vi "get_weather.vi"(4 "Weather Index":u32, 5 "Weather Profiles":refnum<vi>, 6 "error in":errorcluster, 7 "External Weather Control":bool, 9 "simx in":T2={"Config"={"Trajectory"={"Number of frames"=0, "Frame number"=0, "Trajectory"=""}, "Weather"={"id"=""}}, "Connections"={"Simulator Connection"=refnum, "server_ip"="127.0.0.1", "Port"=0, "Sensor connections"=[]}, "Map"={"lanes"={"x"=[], "y"=[], "z"=[]}, "StartPosition"={"start_points"={"locations"=[], "rotations"=[], "type"=[]}, "StartRotation"=[], "StartLocation"=[]}, "Draw Map Size"={"Width"=0, "Height"=0}, "DrawArea"={"min_Y"=0.0, "min_X"=0.0, "Scale X"=0.0, "Scale Y"=0.0}, "Map"=bytes[0], "Map Geojson"=""}}) -> (0 "error out":errorcluster, 1 "Weather Profiles":T9(array[cluster]), 2 "Id":string, 3 "simx out":T2={"Config"={"Trajectory"={"Number of frames"=0, "Frame number"=0, "Trajectory"=""}, "Weather"={"id"=""}}, "Connections"={"Simulator Connection"=refnum, "server_ip"="127.0.0.1", "Port"=0, "Sensor connections"=[]}, "Map"={"lanes"={"x"=[], "y"=[], "z"=[]}, "StartPosition"={"start_points"={"locations"=[], "rotations"=[], "type"=[]}, "StartRotation"=[], "StartLocation"=[]}, "Draw Map Size"={"Width"=0, "Height"=0}, "DrawArea"={"min_Y"=0.0, "min_X"=0.0, "Scale X"=0.0, "Scale Y"=0.0}, "Map"=bytes[0], "Map Geojson"=""}})   [LabVIEW 2025]
doc: "Obtains the weather configuration from a file and populates a cluster with the configuration."
uses:
  controls/simx_connection.ctl
  controls/config.ctl
  controls/trajectory.ctl
  controls/weather.ctl
  controls/connections.ctl
  controls/start_points.ctl
  <vilib>/Utility/miscctls.llb/LVBoundsTypeDef.ctl
  tools/simx_common.vi
panel:
  in  "Cluster":T1
  in  "Weather Configuration":string="{\n \"descriptions\": [\n  {\n   \"CloudColor\": {\n    \"A\": 1.0,\n    \"B\": 1.0,\n    \"G\": 0.9190000295639038,\n    \"R\": 0.8557999730110168\n   },\n   \"CloudOpacity\": 1.1399999856948853,\n   \"Day\": 1,\n   \"FogCutoffDistance\": 0.0,\n   \"FogDensity\": 0.0,\n   \"FogHeightFalloff\": 0.20000000298023224,\n   \"FogInscatteringColor\": {\n    \"A\": 1.0,\n    \"B\": 1.0,\n    \"G\": 0.6380000114440918,\n    \"R\": 0.4449999928474426\n   },\n   \"FogMaxOpacity\": 1.0,\n   \"FogStartDistance\": 0.0,\n   \"HorizonColor\": {\n    \"A\": 1.0,\n    \"B\": 1.0,\n    \"G\": 0.8622000217437744,\n    \"R\": 0.6599000096321106\n   },\n   \"HorizonFalloff\": 10.0,\n   \"Hours\": 12,\n   \"IsDaylightSavingTime\": true,\n   \"Latitude\": 30.237119674682617,\n   \"Longitude\": -97.66307067871094,\n   \"Minutes\": 0,\n   \"Month\": 6,\n   \"NorthOffset\": 0.0,\n   \"OverallSkyColor\": {\n    \"A\": 1.0,\n    \"B\": 1.0,\n    \"G\": 1.0,\n    \"R\": 1.0\n   },\n   \"OverideTimeBasedSunAngle\": false,\n   \"PrecipitationAccumulation\": 0.0,\n   \"PrecipitationAmount\": 0.0,\n   \"PrecipitationType\": \"Rain\",\n   \"SecondFogDensity\": 0.0,\n   \"SecondFogHeightFalloff\": 0.20000000298023224,\n   \"SecondFogHeightOffset\": 0.0,\n   \"Seconds\": 0,\n   \"SkyLightColor\": {\n    \"A\": 0.0,\n    \"B\": 0.1412999927997589,\n    \"G\": 0.1851000040769577,\n    \"R\": 0.19499999284744263\n   },\n   \"SkyLightIntensity\": 1.0,\n   \"StarBrightness\": 3.0,\n   \"SunAzimuthAngle\": 45.0,\n   \"SunBrightness\": 3000.0,\n   \"SunDirectionalLightColor\": {\n    \"A\": 1.0,\n    \"B\": 194.0,\n    \"G\": 239.0,\n    \"R\": 255.0\n   },\n   \"SunDirectionalLightIntensity\": 3.0,\n   \"SunPolarAngle\": 45.0,\n   \"TimeZone\": -5.0,\n   \"WindAngle\": 0.0,\n   \"WindIntensity\": 20.0,\n   \"Year\": 2022,\n   \"ZenithColor\": {\n    \"A\": 1.0,\n    \"B\": 0.29499998688697815,\n    \"G\": 0.10920000076293945,\n    \"R\": 0.03400000184774399\n   },\n   \"bPrecipitation\": false,\n   \"bWind\": false,\n   \"id\": \"Default\"\n  },\n  {\n   \"CloudColor\": {\n    \"A\": 1.0,\n    \"B\": 1.0,\n    \"G\": 0.9190000295639038,\n    \"R\": 0.8557999730110168\n   },\n   \"CloudOpacity\": 0.4285709857940674,\n   \"Day\": 1,\n   \"FogCutoffDistance\": 0.0,\n   \"FogDensity\": 0.007000000216066837,\n   \"FogHeightFalloff\": 1.0671329498291016,\n   \"FogInscatteringColor\": {\n    \"A\": 1.0,\n    \"B\": 1.0,\n    \"G\": 0.6380000114440918,\n    \"R\": 0.4449999928474426\n   },\n   \"FogMaxOpacity\": 1.0,\n   \"FogStartDistance\": 0.0,\n   \"HorizonColor\": {\n    \"A\": 1.0,\n    \"B\": 1.0,\n    \"G\": 0.8622000217437744,\n    \"R\": 0.6599000096321106\n   },\n   \"HorizonFalloff\": 14.28571605682373,\n   \"Hours\": 12,\n   \"IsDaylightSavingTime\": true,\n   \"Latitude\": 30.237119674682617,\n   \"Longitude\": -97.66307067871094,\n   \"Minutes\": 0,\n   \"Month\": 6,\n   \"NorthOffset\": 0.0,\n   \"OverallSkyColor\": {\n    \"A\": 1.0,\n    \"B\": 1.0,\n    \"G\": 1.0,\n    \"R\": 1.0\n   },\n   \"OverideTimeBasedSunAngle\": false,\n   \"PrecipitationAccumulation\": 0.0,\n   \"PrecipitationAmount\": 0.0,\n   \"PrecipitationType\": \"Rain\",\n   \"SecondFogDensity\": 0.0,\n   \"SecondFogHeightFalloff\": 0.3436860144138336,\n   \"SecondFogHeightOffset\": -0.12381000071763992,\n   \"Seconds\": 0,\n   \"SkyLightColor\": {\n    \"A\": 0.0,\n    \"B\": 0.1412999927997589,\n    \"G\": 0.1851000040769577,\n    \"R\": 0.19499999284744263\n   },\n   \"SkyLightIntensity\": 0.5,\n   \"StarBrightness\": 3.0,\n   \"SunAzimuthAngle\": 45.0,\n   \"SunBrightness\": 3000.0,\n   \"SunDirectionalLightColor\": {\n    \"A\": 1.0,\n    \"B\": 1.0,\n    \"G\": 1.0,\n    \"R\": 1.0\n   },\n   \"SunDirectionalLightIntensity\": 3.0,\n   \"SunPolarAngle\": 45.0,\n   \"TimeZone\": -5.0,\n   \"WindAngle\": 0.0,\n   \"WindIntensity\": 20.0,\n   \"Year\": 2022,\n   \"ZenithColor\": {\n    \"A\": 1.0,\n    \"B\": 0.29499998688697815,\n    \"G\": 0.10920000076293945,\n    \"R\": 0.03400000184774399\n   },\n   \"bPrecipitation\": false,\n   \"bWind\": false,\n   \"id\": \"ClearNoon\"\n  },\n  {\n   \"CloudColor\": {\n    \"A\": 1.0,\n    \"B\": 0.05208300054073334,\n    \"G\": 0.05208300054073334,\n    \"R\": 0.05208300054073334\n   },\n   \"CloudOpacity\": 4.0,\n   \"Day\": 1,\n   \"FogCutoffDistance\": 0.0,\n   \"FogDensity\": 0.009999999776482582,\n   \"FogHeightFalloff\": 0.20000000298023224,\n   \"FogInscatteringColor\": {\n    \"A\": 1.0,\n    \"B\": 0.49479201436042786,\n    \"G\": 0.47966399788856506,\n    \"R\": 0.4715990126132965\n   },\n   \"FogMaxOpacity\": 1.0,\n   \"FogStartDistance\": 0.0,\n   \"HorizonColor\": {\n    \"A\": 1.0,\n    \"B\": 0.20000000298023224,\n    \"G\": 0.18744300305843353,\n    \"R\": 0.16899999976158142\n   },\n   \"HorizonFalloff\": 0.0,\n   \"Hours\": 14,\n   \"IsDaylightSavingTime\": true,\n   \"Latitude\": 30.237119674682617,\n   \"Longitude\": -97.66307067871094,\n   \"Minutes\": 0,\n   \"Month\": 6,\n   \"NorthOffset\": 0.0,\n   \"OverallSkyColor\": {\n    \"A\": 1.0,\n    \"B\": 1.0,\n    \"G\": 1.0,\n    \"R\": 1.0\n   },\n   \"OverideTimeBasedSunAngle\": false,\n   \"PrecipitationAccumulation\": 0.0,\n   \"PrecipitationAmount\": 0.0,\n   \"PrecipitationType\": \"Rain\",\n   \"SecondFogDensity\": 0.0,\n   \"SecondFogHeightFalloff\": 0.20000000298023224,\n   \"SecondFogHeightOffset\": 0.0,\n   \"Seconds\": 0,\n   \"SkyLightColor\": {\n    \"A\": 0.0,\n    \"B\": 0.14499999582767487,\n    \"G\": 0.10680299997329712,\n    \"R\": 0.1008870005607605\n   },\n   \"SkyLightIntensity\": 0.5,\n   \"StarBrightness\": 3.0,\n   \"SunAzimuthAngle\": 45.0,\n   \"SunBrightness\": 3000.0,\n   \"SunDirectionalLightColor\": {\n    \"A\": 1.0,\n    \"B\": 0.25520798563957214,\n    \"G\": 0.25520798563957214,\n    \"R\": 0.25520798563957214\n   },\n   \"SunDirectionalLightIntensity\": 3.0,\n   \"SunPolarAngle\": 45.0,\n   \"TimeZone\": -5.0,\n   \"WindAngle\": 0.0,\n   \"WindIntensity\": 20.0,\n   \"Year\": 2022,\n   \"ZenithColor\": {\n    \"A\": 1.0,\n    \"B\": 0.29499998688697815,\n    \"G\": 0.1812479943037033,\n    \"R\": 0.13520799577236176\n   },\n   \"bPrecipitation\": false,\n   \"bWind\": false,\n   \"id\": \"CloudyNoon\"\n  },\n  {\n   \"CloudColor\": {\n    \"A\": 1.0,\n    \"B\": 0.1899999976158142,\n    \"G\": 0.15923500061035156,\n    \"R\": 0.14362700283527374\n   },\n   \"CloudOpacity\": 1.5714290142059326,\n   \"Day\": 1,\n   \"FogCutoffDistance\": 0.0,\n   \"FogDensity\": 0.005237999837845564,\n   \"FogHeightFalloff\": 0.20000000298023224,\n   \"FogInscatteringColor\": {\n    \"A\": 1.0,\n    \"B\": 1.0,\n    \"G\": 0.6380000114440918,\n    \"R\": 0.4449999928474426\n   },\n   \"FogMaxOpacity\": 0.028571000322699547,\n   \"FogStartDistance\": 0.0,\n   \"HorizonColor\": {\n    \"A\": 1.0,\n    \"B\": 0.6299999952316284,\n    \"G\": 0.5904449820518494,\n    \"R\": 0.5323500037193298\n   },\n   \"HorizonFalloff\": 10.476192474365234,\n   \"Hours\": 12,\n   \"IsDaylightSavingTime\": true,\n   \"Latitude\": 30.237119674682617,\n   \"Longitude\": -97.66307067871094,\n   \"Minutes\": 0,\n   \"Month\": 6,\n   \"NorthOffset\": 0.0,\n   \"OverallSkyColor\": {\n    \"A\": 1.0,\n    \"B\": 0.5181000232696533,\n    \"G\": 0.6304129958152771,\n    \"R\": 0.6600000262260437\n   },\n   \"OverideTimeBasedSunAngle\": false,\n   \"PrecipitationAccumulation\": 28.57143211364746,\n   \"PrecipitationAmount\": 0.0,\n   \"PrecipitationType\": \"Rain\",\n   \"SecondFogDensity\": 0.001429000054486096,\n   \"SecondFogHeightFalloff\": 2.0,\n   \"SecondFogHeightOffset\": 0.3131600022315979,\n   \"Seconds\": 0,\n   \"SkyLightColor\": {\n    \"A\": 0.0,\n    \"B\": 0.07559999823570251,\n    \"G\": 0.12014999985694885,\n    \"R\": 0.13500000536441803\n   },\n   \"SkyLightIntensity\": 1.0,\n   \"StarBrightness\": 3.0,\n   \"SunAzimuthAngle\": 45.0,\n   \"SunBrightness\": 0.0,\n   \"SunDirectionalLightColor\": {\n    \"A\": 1.0,\n    \"B\": 1.0,\n    \"G\": 1.0,\n    \"R\": 1.0\n   },\n   \"SunDirectionalLightIntensity\": 3.0,\n   \"SunPolarAngle\": 45.0,\n   \"TimeZone\": -5.0,\n   \"WindAngle\": 0.0,\n   \"WindIntensity\": 20.0,\n   \"Year\": 2022,\n   \"ZenithColor\": {\n    \"A\": 1.0,\n    \"B\": 0.29499998688697815,\n    \"G\": 0.10920000076293945,\n    \"R\": 0.03400000184774399\n   },\n   \"bPrecipitation\": true,\n   \"bWind\": false,\n   \"id\": \"WetNoon\"\n  },\n  {\n   \"CloudColor\": {\n    \"A\": 1.0,\n    \"B\": 0.27164098620414734,\n    \"G\": 0.3050000071525574,\n    \"R\": 0.2995159924030304\n   },\n   \"CloudOpacity\": 1.0,\n   \"Day\": 1,\n   \"FogCutoffDistance\": 0.0,\n   \"FogDensity\": 0.009523999877274036,\n   \"FogHeightFalloff\": 0.20000000298023224,\n   \"FogInscatteringColor\": {\n    \"A\": 1.0,\n    \"B\": 1.0,\n    \"G\": 0.8581939935684204,\n    \"R\": 0.548704981803894\n   },\n   \"FogMaxOpacity\": 1.0,\n   \"FogStartDistance\": 0.0,\n   \"HorizonColor\": {\n    \"A\": 1.0,\n    \"B\": 0.0,\n    \"G\": 0.0,\n    \"R\": 0.0\n   },\n   \"HorizonFalloff\": 3.0,\n   \"Hours\": 12,\n   \"IsDaylightSavingTime\": true,\n   \"Latitude\": 30.237119674682617,\n   \"Longitude\": -97.66307067871094,\n   \"Minutes\": 0,\n   \"Month\": 6,\n   \"NorthOffset\": 0.0,\n   \"OverallSkyColor\": {\n    \"A\": 1.0,\n    \"B\": 0.5181000232696533,\n    \"G\": 0.6304129958152771,\n    \"R\": 0.6600000262260437\n   },\n   \"OverideTimeBasedSunAngle\": false,\n   \"PrecipitationAccumulation\": 47.70600128173828,\n   \"PrecipitationAmount\": 0.0,\n   \"PrecipitationType\": \"Rain\",\n   \"SecondFogDensity\": 0.0,\n   \"SecondFogHeightFalloff\": 0.20000000298023224,\n   \"SecondFogHeightOffset\": 0.0,\n   \"Seconds\": 0,\n   \"SkyLightColor\": {\n    \"A\": 0.0,\n    \"B\": 0.1267089992761612,\n    \"G\": 0.13369999825954437,\n    \"R\": 0.140625\n   },\n   \"SkyLightIntensity\": 1.0,\n   \"StarBrightness\": 3.0,\n   \"SunAzimuthAngle\": 174.0,\n   \"SunBrightness\": 0.0,\n   \"SunDirectionalLightColor\": {\n    \"A\": 1.0,\n    \"B\": 0.20507900416851044,\n    \"G\": 0.30498701333999634,\n    \"R\": 0.2874409854412079\n   },\n   \"SunDirectionalLightIntensity\": 1.8350000381469727,\n   \"SunPolarAngle\": 174.0,\n   \"TimeZone\": -5.0,\n   \"WindAngle\": 0.0,\n   \"WindIntensity\": 20.0,\n   \"Year\": 2018,\n   \"ZenithColor\": {\n    \"A\": 1.0,\n    \"B\": 1.0,\n    \"G\": 1.0,\n    \"R\": 1.0\n   },\n   \"bPrecipitation\": true,\n   \"bWind\": false,\n   \"id\": \"WetCloudyNoon\"\n  },\n  {\n   \"CloudColor\": {\n    \"A\": 1.0,\n    \"B\": 0.05000000074505806,\n    \"G\": 0.04594999924302101,\n    \"R\": 0.042789001017808914\n   },\n   \"CloudOpacity\": 1.0,\n   \"Day\": 1,\n   \"FogCutoffDistance\": 0.0,\n   \"FogDensity\": 0.008570999838411808,\n   \"FogHeightFalloff\": 0.20000000298023224,\n   \"FogInscatteringColor\": {\n    \"A\": 1.0,\n    \"B\": 0.4889959990978241,\n    \"G\": 0.6769369840621948,\n    \"R\": 0.7395830154418945\n   },\n   \"FogMaxOpacity\": 1.0,\n   \"FogStartDistance\": 0.0,\n   \"HorizonColor\": {\n    \"A\": 1.0,\n    \"B\": 0.20000000298023224,\n    \"G\": 0.18744300305843353,\n    \"R\": 0.16899999976158142\n   },\n   \"HorizonFalloff\": 3.0,\n   \"Hours\": 12,\n   \"IsDaylightSavingTime\": true,\n   \"Latitude\": 30.237119674682617,\n   \"Longitude\": -97.66307067871094,\n   \"Minutes\": 0,\n   \"Month\": 6,\n   \"NorthOffset\": 0.0,\n   \"OverallSkyColor\": {\n    \"A\": 1.0,\n    \"B\": 1.0,\n    \"G\": 1.0,\n    \"R\": 1.0\n   },\n   \"OverideTimeBasedSunAngle\": false,\n   \"PrecipitationAccumulation\": 50.0,\n   \"PrecipitationAmount\": 40.0,\n   \"PrecipitationType\": \"Rain\",\n   \"SecondFogDensity\": 0.0,\n   \"SecondFogHeightFalloff\": 0.20000000298023224,\n   \"SecondFogHeightOffset\": 0.0,\n   \"Seconds\": 0,\n   \"SkyLightColor\": {\n    \"A\": 0.0,\n    \"B\": 0.17000000178813934,\n    \"G\": 0.12155699729919434,\n    \"R\": 0.1198820024728775\n   },\n   \"SkyLightIntensity\": 1.0,\n   \"StarBrightness\": 3.0,\n   \"SunAzimuthAngle\": 45.0,\n   \"SunBrightness\": 3000.0,\n   \"SunDirectionalLightColor\": {\n    \"A\": 1.0,\n    \"B\": 1.0,\n    \"G\": 1.0,\n    \"R\": 1.0\n   },\n   \"SunDirectionalLightIntensity\": 3.0,\n   \"SunPolarAngle\": 45.0,\n   \"TimeZone\": -5.0,\n   \"WindAngle\": -80.0,\n   \"WindIntensity\": 40.0,\n   \"Year\": 2022,\n   \"ZenithColor\": {\n    \"A\": 1.0,\n    \"B\": 0.3700000047683716,\n    \"G\": 0.3700000047683716,\n    \"R\": 0.3700000047683716\n   },\n   \"bPrecipitation\": true,\n   \"bWind\": true,\n   \"id\": \"MidRainyNoon\"\n  },\n  {\n   \"CloudColor\": {\n    \"A\": 1.0,\n    \"B\": 0.046875,\n    \"G\": 0.04307800158858299,\n    \"R\": 0.04011499881744385\n   },\n   \"CloudOpacity\": 1.0,\n   \"Day\": 1,\n   \"FogCutoffDistance\": 0.0,\n   \"FogDensity\": 0.0042860000394284725,\n   \"FogHeightFalloff\": 0.4007999897003174,\n   \"FogInscatteringColor\": {\n    \"A\": 1.0,\n    \"B\": 1.0,\n    \"G\": 0.6380000114440918,\n    \"R\": 0.4449999928474426\n   },\n   \"FogMaxOpacity\": 0.5904759764671326,\n   \"FogStartDistance\": 0.0,\n   \"HorizonColor\": {\n    \"A\": 1.0,\n    \"B\": 0.11458300054073334,\n    \"G\": 0.10738900303840637,\n    \"R\": 0.09682299941778183\n   },\n   \"HorizonFalloff\": 3.0,\n   \"Hours\": 12,\n   \"IsDaylightSavingTime\": true,\n   \"Latitude\": 30.237119674682617,\n   \"Longitude\": -97.66307067871094,\n   \"Minutes\": 0,\n   \"Month\": 6,\n   \"NorthOffset\": 0.0,\n   \"OverallSkyColor\": {\n    \"A\": 1.0,\n    \"B\": 0.23455099761486053,\n    \"G\": 0.18782100081443787,\n    \"R\": 0.15592600405216217\n   },\n   \"OverideTimeBasedSunAngle\": false,\n   \"PrecipitationAccumulation\": 87.24800109863281,\n   \"PrecipitationAmount\": 80.0,\n   \"PrecipitationType\": \"Rain\",\n   \"SecondFogDensity\": 0.010475999675691128,\n   \"SecondFogHeightFalloff\": 1.1899809837341309,\n   \"SecondFogHeightOffset\": 0.6190469861030579,\n   \"Seconds\": 0,\n   \"SkyLightColor\": {\n    \"A\": 0.0,\n    \"B\": 0.18000000715255737,\n    \"G\": 0.12870700657367706,\n    \"R\": 0.1269340068101883\n   },\n   \"SkyLightIntensity\": 1.0,\n   \"StarBrightness\": 3.0,\n   \"SunAzimuthAngle\": 45.0,\n   \"SunBrightness\": 0.0,\n   \"SunDirectionalLightColor\": {\n    \"A\": 1.0,\n    \"B\": 0.203125,\n    \"G\": 0.1996610015630722,\n    \"R\": 0.1996610015630722\n   },\n   \"SunDirectionalLightIntensity\": 3.0,\n   \"SunPolarAngle\": 45.0,\n   \"TimeZone\": -5.0,\n   \"WindAngle\": -60.0,\n   \"WindIntensity\": 39.0476188659668,\n   \"Year\": 2022,\n   \"ZenithColor\": {\n    \"A\": 1.0,\n    \"B\": 0.5799999833106995,\n    \"G\": 0.5799999833106995,\n    \"R\": 0.5799999833106995\n   },\n   \"bPrecipitation\": true,\n   \"bWind\": true,\n   \"id\": \"HardRainNoon\"\n  },\n  {\n   \"CloudColor\": {\n    \"A\": 1.0,\n    \"B\": 0.18229199945926666,\n    \"G\": 0.1675260066986084,\n    \"R\": 0.1560010015964508\n   },\n   \"CloudOpacity\": 1.0,\n   \"Day\": 1,\n   \"FogCutoffDistance\": 0.0,\n   \"FogDensity\": 0.03333299979567528,\n   \"FogHeightFalloff\": 0.20000000298023224,\n   \"FogInscatteringColor\": {\n    \"A\": 1.0,\n    \"B\": 0.375,\n    \"G\": 0.3648090064525604,\n    \"R\": 0.359375\n   },\n   \"FogMaxOpacity\": 1.0,\n   \"FogStartDistance\": 0.0,\n   \"HorizonColor\": {\n    \"A\": 1.0,\n    \"B\": 0.20000000298023224,\n    \"G\": 0.18744300305843353,\n    \"R\": 0.16899999976158142\n   },\n   \"HorizonFalloff\": 3.0,\n   \"Hours\": 10,\n   \"IsDaylightSavingTime\": true,\n   \"Latitude\": 30.237119674682617,\n   \"Longitude\": -97.66307067871094,\n   \"Minutes\": 0,\n   \"Month\": 6,\n   \"NorthOffset\": 0.0,\n   \"OverallSkyColor\": {\n    \"A\": 1.0,\n    \"B\": 1.0,\n    \"G\": 1.0,\n    \"R\": 1.0\n   },\n   \"OverideTimeBasedSunAngle\": false,\n   \"PrecipitationAccumulation\": 61.926998138427734,\n   \"PrecipitationAmount\": 10.550000190734863,\n   \"PrecipitationType\": \"Rain\",\n   \"SecondFogDensity\": 0.018571000546216965,\n   \"SecondFogHeightFalloff\": 0.20000000298023224,\n   \"SecondFogHeightOffset\": 0.0,\n   \"Seconds\": 0,\n   \"SkyLightColor\": {\n    \"A\": 0.0,\n    \"B\": 0.07291699945926666,\n    \"G\": 0.07291699945926666,\n    \"R\": 0.07291699945926666\n   },\n   \"SkyLightIntensity\": 0.5,\n   \"StarBrightness\": 3.0,\n   \"SunAzimuthAngle\": 45.0,\n   \"SunBrightness\": 3000.0,\n   \"SunDirectionalLightColor\": {\n    \"A\": 1.0,\n    \"B\": 1.0,\n    \"G\": 1.0,\n    \"R\": 1.0\n   },\n   \"SunDirectionalLightIntensity\": 1.5,\n   \"SunPolarAngle\": 45.0,\n   \"TimeZone\": -5.0,\n   \"WindAngle\": 20.0,\n   \"WindIntensity\": 10.0,\n   \"Year\": 2022,\n   \"ZenithColor\": {\n    \"A\": 1.0,\n    \"B\": 0.0,\n    \"G\": 0.0,\n    \"R\": 0.0\n   },\n   \"bPrecipitation\": true,\n   \"bWind\": true,\n   \"id\": \"SoftRainNoon\"\n  },\n  {\n   \"CloudColor\": {\n    \"A\": 1.0,\n    \"B\": 0.08333300054073334,\n    \"G\": 0.5042790174484253,\n    \"R\": 1.0\n   },\n   \"CloudOpacity\": 0.5714290142059326,\n   \"Day\": 1,\n   \"FogCutoffDistance\": 0.0,\n   \"FogDensity\": 0.003000000026077032,\n   \"FogHeightFalloff\": 0.20000000298023224,\n   \"FogInscatteringColor\": {\n    \"A\": 1.0,\n    \"B\": 0.4279409945011139,\n    \"G\": 0.7066850066184998,\n    \"R\": 0.8470590114593506\n   },\n   \"FogMaxOpacity\": 1.0,\n   \"FogStartDistance\": 2800.0,\n   \"HorizonColor\": {\n    \"A\": 1.0,\n    \"B\": 0.04664900153875351,\n    \"G\": 0.2190060019493103,\n    \"R\": 0.7450000047683716\n   },\n   \"HorizonFalloff\": 3.0,\n   \"Hours\": 19,\n   \"IsDaylightSavingTime\": true,\n   \"Latitude\": 30.237119674682617,\n   \"Longitude\": -97.66307067871094,\n   \"Minutes\": 0,\n   \"Month\": 6,\n   \"NorthOffset\": 0.0,\n   \"OverallSkyColor\": {\n    \"A\": 1.0,\n    \"B\": 1.0,\n    \"G\": 1.0,\n    \"R\": 1.0\n   },\n   \"OverideTimeBasedSunAngle\": false,\n   \"PrecipitationAccumulation\": 0.0,\n   \"PrecipitationAmount\": 0.0,\n   \"PrecipitationType\": \"Rain\",\n   \"SecondFogDensity\": 0.0020000000949949026,\n   \"SecondFogHeightFalloff\": 0.6000000238418579,\n   \"SecondFogHeightOffset\": 0.0,\n   \"Seconds\": 0,\n   \"SkyLightColor\": {\n    \"A\": 0.0,\n    \"B\": 0.109375,\n    \"G\": 0.07472400367259979,\n    \"R\": 0.07621999830007553\n   },\n   \"SkyLightIntensity\": 1.0,\n   \"StarBrightness\": 3.0,\n   \"SunAzimuthAngle\": 45.0,\n   \"SunBrightness\": 3000.0,\n   \"SunDirectionalLightColor\": {\n    \"A\": 1.0,\n    \"B\": 0.17010000348091125,\n    \"G\": 0.3474699854850769,\n    \"R\": 0.8100000023841858\n   },\n   \"SunDirectionalLightIntensity\": 3.0,\n   \"SunPolarAngle\": 45.0,\n   \"TimeZone\": -5.0,\n   \"WindAngle\": 0.0,\n   \"WindIntensity\": 20.0,\n   \"Year\": 2022,\n   \"ZenithColor\": {\n    \"A\": 1.0,\n    \"B\": 0.10499999672174454,\n    \"G\": 0.04410000145435333,\n    \"R\": 0.04637499898672104\n   },\n   \"bPrecipitation\": false,\n   \"bWind\": false,\n   \"id\": \"ClearSunset\"\n  },\n  {\n   \"CloudColor\": {\n    \"A\": 1.0,\n    \"B\": 0.13456499576568604,\n    \"G\": 0.20229600369930267,\n    \"R\": 0.5208330154418945\n   },\n   \"CloudOpacity\": 1.4285720586776733,\n   \"Day\": 1,\n   \"FogCutoffDistance\": 0.0,\n   \"FogDensity\": 0.0009519999730400741,\n   \"FogHeightFalloff\": 0.20000000298023224,\n   \"FogInscatteringColor\": {\n    \"A\": 1.0,\n    \"B\": 0.4463469982147217,\n    \"G\": 0.5565620064735413,\n    \"R\": 1.0\n   },\n   \"FogMaxOpacity\": 1.0,\n   \"FogStartDistance\": 0.0,\n   \"HorizonColor\": {\n    \"A\": 1.0,\n    \"B\": 0.09927500039339066,\n    \"G\": 0.18896199762821198,\n    \"R\": 1.0\n   },\n   \"HorizonFalloff\": 3.5,\n   \"Hours\": 19,\n   \"IsDaylightSavingTime\": true,\n   \"Latitude\": 30.237119674682617,\n   \"Longitude\": -97.66307067871094,\n   \"Minutes\": 0,\n   \"Month\": 6,\n   \"NorthOffset\": 0.0,\n   \"OverallSkyColor\": {\n    \"A\": 1.0,\n    \"B\": 0.4099999964237213,\n    \"G\": 0.4099999964237213,\n    \"R\": 0.4099999964237213\n   },\n   \"OverideTimeBasedSunAngle\": false,\n   \"PrecipitationAccumulation\": 0.0,\n   \"PrecipitationAmount\": 0.0,\n   \"PrecipitationType\": \"Rain\",\n   \"SecondFogDensity\": 0.0,\n   \"SecondFogHeightFalloff\": 0.20000000298023224,\n   \"SecondFogHeightOffset\": 0.0,\n   \"Seconds\": 0,\n   \"SkyLightColor\": {\n    \"A\": 0.0,\n    \"B\": 0.27000001072883606,\n    \"G\": 0.19511300325393677,\n    \"R\": 0.19304999709129333\n   },\n   \"SkyLightIntensity\": 1.0,\n   \"StarBrightness\": 3.0,\n   \"SunAzimuthAngle\": 45.0,\n   \"SunBrightness\": 3000.0,\n   \"SunDirectionalLightColor\": {\n    \"A\": 1.0,\n    \"B\": 0.08300299942493439,\n    \"G\": 0.34716200828552246,\n    \"R\": 0.8100000023841858\n   },\n   \"SunDirectionalLightIntensity\": 3.0,\n   \"SunPolarAngle\": 45.0,\n   \"TimeZone\": -5.0,\n   \"WindAngle\": 0.0,\n   \"WindIntensity\": 20.0,\n   \"Year\": 2022,\n   \"ZenithColor\": {\n    \"A\": 1.0,\n    \"B\": 0.10499999672174454,\n    \"G\": 0.04410000145435333,\n    \"R\": 0.04637499898672104\n   },\n   \"bPrecipitation\": false,\n   \"bWind\": false,\n   \"id\": \"CloudySunset\"\n  },\n  {\n   \"CloudColor\": {\n    \"A\": 1.0,\n    \"B\": 0.13563300669193268,\n    \"G\": 0.201555997133255,\n    \"R\": 0.5209959745407104\n   },\n   \"CloudOpacity\": 1.2857149839401245,\n   \"Day\": 1,\n   \"FogCutoffDistance\": 0.0,\n   \"FogDensity\": 0.010475999675691128,\n   \"FogHeightFalloff\": 0.20000000298023224,\n   \"FogInscatteringColor\": {\n    \"A\": 1.0,\n    \"B\": 0.10461600124835968,\n    \"G\": 0.04373500123620033,\n    \"R\": 0.0466650016605854\n   },\n   \"FogMaxOpacity\": 1.0,\n   \"FogStartDistance\": 0.0,\n   \"HorizonColor\": {\n    \"A\": 1.0,\n    \"B\": 0.09989900141954422,\n    \"G\": 0.18782100081443787,\n    \"R\": 1.0\n   },\n   \"HorizonFalloff\": 3.5,\n   \"Hours\": 20,\n   \"IsDaylightSavingTime\": true,\n   \"Latitude\": 30.237119674682617,\n   \"Longitude\": -97.66307067871094,\n   \"Minutes\": 0,\n   \"Month\": 6,\n   \"NorthOffset\": 0.0,\n   \"OverallSkyColor\": {\n    \"A\": 1.0,\n    \"B\": 0.41254299879074097,\n    \"G\": 0.41254299879074097,\n    \"R\": 0.41254299879074097\n   },\n   \"OverideTimeBasedSunAngle\": false,\n   \"PrecipitationAccumulation\": 65.0459976196289,\n   \"PrecipitationAmount\": 0.0,\n   \"PrecipitationType\": \"Rain\",\n   \"SecondFogDensity\": 0.0,\n   \"SecondFogHeightFalloff\": 0.20000000298023224,\n   \"SecondFogHeightOffset\": 0.0,\n   \"Seconds\": 0,\n   \"SkyLightColor\": {\n    \"A\": 0.0,\n    \"B\": 0.20000000298023224,\n    \"G\": 0.10999999940395355,\n    \"R\": 0.1138869971036911\n   },\n   \"SkyLightIntensity\": 1.0,\n   \"StarBrightness\": 3.0,\n   \"SunAzimuthAngle\": 174.0,\n   \"SunBrightness\": 3000.0,\n   \"SunDirectionalLightColor\": {\n    \"A\": 1.0,\n    \"B\": 0.08300299942493439,\n    \"G\": 0.34716200828552246,\n    \"R\": 0.8100000023841858\n   },\n   \"SunDirectionalLightIntensity\": 3.0,\n   \"SunPolarAngle\": 174.0,\n   \"TimeZone\": -5.0,\n   \"WindAngle\": 0.0,\n   \"WindIntensity\": 20.0,\n   \"Year\": 2022,\n   \"ZenithColor\": {\n    \"A\": 1.0,\n    \"B\": 0.10499999672174454,\n    \"G\": 0.04410000145435333,\n    \"R\": 0.04637499898672104\n   },\n   \"bPrecipitation\": true,\n   \"bWind\": false,\n   \"id\": \"WetSunset\"\n  },\n  {\n   \"CloudColor\": {\n    \"A\": 1.0,\n    \"B\": 0.13563300669193268,\n    \"G\": 0.201555997133255,\n    \"R\": 0.5209959745407104\n   },\n   \"CloudOpacity\": 1.8571430444717407,\n   \"Day\": 1,\n   \"FogCutoffDistance\": 0.0,\n   \"FogDensity\": 0.0,\n   \"FogHeightFalloff\": 0.20000000298023224,\n   \"FogInscatteringColor\": {\n    \"A\": 1.0,\n    \"B\": 1.0,\n    \"G\": 0.6380000114440918,\n    \"R\": 0.4449999928474426\n   },\n   \"FogMaxOpacity\": 1.0,\n   \"FogStartDistance\": 0.0,\n   \"HorizonColor\": {\n    \"A\": 1.0,\n    \"B\": 0.17464199662208557,\n    \"G\": 0.21405300498008728,\n    \"R\": 0.578125\n   },\n   \"HorizonFalloff\": 5.0,\n   \"Hours\": 19,\n   \"IsDaylightSavingTime\": true,\n   \"Latitude\": 30.237119674682617,\n   \"Longitude\": -97.66307067871094,\n   \"Minutes\": 0,\n   \"Month\": 6,\n   \"NorthOffset\": 0.0,\n   \"OverallSkyColor\": {\n    \"A\": 1.0,\n    \"B\": 0.26041701436042786,\n    \"G\": 0.26041701436042786,\n    \"R\": 0.26041701436042786\n   },\n   \"OverideTimeBasedSunAngle\": false,\n   \"PrecipitationAccumulation\": 25.71428680419922,\n   \"PrecipitationAmount\": 0.0,\n   \"PrecipitationType\": \"Rain\",\n   \"SecondFogDensity\": 0.0,\n   \"SecondFogHeightFalloff\": 0.20000000298023224,\n   \"SecondFogHeightOffset\": 0.0,\n   \"Seconds\": 0,\n   \"SkyLightColor\": {\n    \"A\": 1.0,\n    \"B\": 0.15625,\n    \"G\": 0.1124190017580986,\n    \"R\": 0.1124190017580986\n   },\n   \"SkyLightIntensity\": 1.0,\n   \"StarBrightness\": 3.0,\n   \"SunAzimuthAngle\": 45.0,\n   \"SunBrightness\": 3000.0,\n   \"SunDirectionalLightColor\": {\n    \"A\": 1.0,\n    \"B\": 0.08300299942493439,\n    \"G\": 0.34716200828552246,\n    \"R\": 0.8100000023841858\n   },\n   \"SunDirectionalLightIntensity\": 3.0,\n   \"SunPolarAngle\": 45.0,\n   \"TimeZone\": -5.0,\n   \"WindAngle\": 0.0,\n   \"WindIntensity\": 20.0,\n   \"Year\": 2022,\n   \"ZenithColor\": {\n    \"A\": 1.0,\n    \"B\": 0.10499999672174454,\n    \"G\": 0.04410000145435333,\n    \"R\": 0.04637499898672104\n   },\n   \"bPrecipitation\": true,\n   \"bWind\": false,\n   \"id\": \"WetCloudySunset\"\n  },\n  {\n   \"CloudColor\": {\n    \"A\": 1.0,\n    \"B\": 0.13563300669193268,\n    \"G\": 0.201555997133255,\n    \"R\": 0.5209959745407104\n   },\n   \"CloudOpacity\": 2.9285709857940674,\n   \"Day\": 1,\n   \"FogCutoffDistance\": 0.0,\n   \"FogDensity\": 0.008094999939203262,\n   \"FogHeightFalloff\": 0.20000000298023224,\n   \"FogInscatteringColor\": {\n    \"A\": 1.0,\n    \"B\": 0.2620440125465393,\n    \"G\": 0.32677599787712097,\n    \"R\": 0.359375\n   },\n   \"FogMaxOpacity\": 1.0,\n   \"FogStartDistance\": 0.0,\n   \"HorizonColor\": {\n    \"A\": 1.0,\n    \"B\": 0.09989900141954422,\n    \"G\": 0.18782100081443787,\n    \"R\": 1.0\n   },\n   \"HorizonFalloff\": 3.0,\n   \"Hours\": 20,\n   \"IsDaylightSavingTime\": true,\n   \"Latitude\": 30.237119674682617,\n   \"Longitude\": -97.66307067871094,\n   \"Minutes\": 0,\n   \"Month\": 6,\n   \"NorthOffset\": 0.0,\n   \"OverallSkyColor\": {\n    \"A\": 1.0,\n    \"B\": 0.41254299879074097,\n    \"G\": 0.41254299879074097,\n    \"R\": 0.41254299879074097\n   },\n   \"OverideTimeBasedSunAngle\": false,\n   \"PrecipitationAccumulation\": 88.072998046875,\n   \"PrecipitationAmount\": 37.15599822998047,\n   \"PrecipitationType\": \"Rain\",\n   \"SecondFogDensity\": 0.0,\n   \"SecondFogHeightFalloff\": 0.20000000298023224,\n   \"SecondFogHeightOffset\": 0.0,\n   \"Seconds\": 0,\n   \"SkyLightColor\": {\n    \"A\": 0.0,\n    \"B\": 0.04906199872493744,\n    \"G\": 0.0642710030078888,\n    \"R\": 0.06770800054073334\n   },\n   \"SkyLightIntensity\": 1.0,\n   \"StarBrightness\": 3.0,\n   \"SunAzimuthAngle\": 45.0,\n   \"SunBrightness\": 3000.0,\n   \"SunDirectionalLightColor\": {\n    \"A\": 1.0,\n    \"B\": 0.08300299942493439,\n    \"G\": 0.34716200828552246,\n    \"R\": 0.8100000023841858\n   },\n   \"SunDirectionalLightIntensity\": 3.0,\n   \"SunPolarAngle\": 45.0,\n   \"TimeZone\": -5.0,\n   \"WindAngle\": 0.0,\n   \"WindIntensity\": 20.0,\n   \"Year\": 2022,\n   \"ZenithColor\": {\n    \"A\": 1.0,\n    \"B\": 0.10461600124835968,\n    \"G\": 0.04373500123620033,\n    \"R\": 0.0466650016605854\n   },\n   \"bPrecipitation\": true,\n   \"bWind\": false,\n   \"id\": \"MidRainSunset\"\n  },\n  {\n   \"CloudColor\": {\n    \"A\": 1.0,\n    \"B\": 0.09895800054073334,\n    \"G\": 0.09895800054073334,\n    \"R\": 0.09895800054073334\n   },\n   \"CloudOpacity\": 4.0,\n   \"Day\": 1,\n   \"FogCutoffDistance\": 0.0,\n   \"FogDensity\": 0.005237999837845564,\n   \"FogHeightFalloff\": 0.6378759741783142,\n   \"FogInscatteringColor\": {\n    \"A\": 1.0,\n    \"B\": 0.4017229974269867,\n    \"G\": 0.5206969976425171,\n    \"R\": 0.5208330154418945\n   },\n   \"FogMaxOpacity\": 1.0,\n   \"FogStartDistance\": 0.0,\n   \"HorizonColor\": {\n    \"A\": 1.0,\n    \"B\": 0.08420199900865555,\n    \"G\": 0.10953900218009949,\n    \"R\": 0.16666699945926666\n   },\n   \"HorizonFalloff\": 3.0,\n   \"Hours\": 20,\n   \"IsDaylightSavingTime\": true,\n   \"Latitude\": 30.237119674682617,\n   \"Longitude\": -97.66307067871094,\n   \"Minutes\": 0,\n   \"Month\": 6,\n   \"NorthOffset\": 0.0,\n   \"OverallSkyColor\": {\n    \"A\": 1.0,\n    \"B\": 0.08333300054073334,\n    \"G\": 0.1035889983177185,\n    \"R\": 0.125\n   },\n   \"OverideTimeBasedSunAngle\": false,\n   \"PrecipitationAccumulation\": 100.0,\n   \"PrecipitationAmount\": 84.86199951171875,\n   \"PrecipitationType\": \"Rain\",\n   \"SecondFogDensity\": 0.0,\n   \"SecondFogHeightFalloff\": 0.20000000298023224,\n   \"SecondFogHeightOffset\": 0.0,\n   \"Seconds\": 0,\n   \"SkyLightColor\": {\n    \"A\": 0.0,\n    \"B\": 0.25,\n    \"G\": 0.3833560049533844,\n    \"R\": 0.5\n   },\n   \"SkyLightIntensity\": 0.20000000298023224,\n   \"StarBrightness\": 3.0,\n   \"SunAzimuthAngle\": 45.0,\n   \"SunBrightness\": 3000.0,\n   \"SunDirectionalLightColor\": {\n    \"A\": 1.0,\n    \"B\": 0.046929001808166504,\n    \"G\": 0.04880199953913689,\n    \"R\": 0.05208300054073334\n   },\n   \"SunDirectionalLightIntensity\": 0.0,\n   \"SunPolarAngle\": 45.0,\n   \"TimeZone\": -5.0,\n   \"WindAngle\": 0.0,\n   \"WindIntensity\": 20.0,\n   \"Year\": 2022,\n   \"ZenithColor\": {\n    \"A\": 1.0,\n    \"B\": 0.17773400247097015,\n    \"G\": 0.17977400124073029,\n    \"R\": 0.1875\n   },\n   \"bPrecipitation\": true,\n   \"bWind\": false,\n   \"id\": \"HardRainSunset\"\n  },\n  {\n   \"CloudColor\": {\n    \"A\": 1.0,\n    \"B\": 0.04177499935030937,\n    \"G\": 0.04890099912881851,\n    \"R\": 0.05729199945926666\n   },\n   \"CloudOpacity\": 3.0,\n   \"Day\": 1,\n   \"FogCutoffDistance\": 0.0,\n   \"FogDensity\": 0.0061900001019239426,\n   \"FogHeightFalloff\": 0.20000000298023224,\n   \"FogInscatteringColor\": {\n    \"A\": 1.0,\n    \"B\": 0.6029350161552429,\n    \"G\": 0.6328070163726807,\n    \"R\": 1.0\n   },\n   \"FogMaxOpacity\": 0.028571000322699547,\n   \"FogStartDistance\": 5000.0,\n   \"HorizonColor\": {\n    \"A\": 1.0,\n    \"B\": 0.0,\n    \"G\": 0.3595309853553772,\n    \"R\": 0.609375\n   },\n   \"HorizonFalloff\": 1.8350000381469727,\n   \"Hours\": 20,\n   \"IsDaylightSavingTime\": true,\n   \"Latitude\": 30.237119674682617,\n   \"Longitude\": -97.66307067871094,\n   \"Minutes\": 0,\n   \"Month\": 6,\n   \"NorthOffset\": 0.0,\n   \"OverallSkyColor\": {\n    \"A\": 1.0,\n    \"B\": 0.1875,\n    \"G\": 0.1875,\n    \"R\": 0.1875\n   },\n   \"OverideTimeBasedSunAngle\": false,\n   \"PrecipitationAccumulation\": 53.21099853515625,\n   \"PrecipitationAmount\": 8.715999603271484,\n   \"PrecipitationType\": \"Rain\",\n   \"SecondFogDensity\": 0.0,\n   \"SecondFogHeightFalloff\": 0.20000000298023224,\n   \"SecondFogHeightOffset\": 0.0,\n   \"Seconds\": 0,\n   \"SkyLightColor\": {\n    \"A\": 0.0,\n    \"B\": 0.07080399990081787,\n    \"G\": 0.08194799721240997,\n    \"R\": 0.09895800054073334\n   },\n   \"SkyLightIntensity\": 1.0,\n   \"StarBrightness\": 3.0,\n   \"SunAzimuthAngle\": 45.0,\n   \"SunBrightness\": 3000.0,\n   \"SunDirectionalLightColor\": {\n    \"A\": 1.0,\n    \"B\": 0.08300299942493439,\n    \"G\": 0.34716200828552246,\n    \"R\": 0.8100000023841858\n   },\n   \"SunDirectionalLightIntensity\": 3.0,\n   \"SunPolarAngle\": 45.0,\n   \"TimeZone\": -5.0,\n   \"WindAngle\": 0.0,\n   \"WindIntensity\": 20.0,\n   \"Year\": 2022,\n   \"ZenithColor\": {\n    \"A\": 1.0,\n    \"B\": 0.20507900416851044,\n    \"G\": 0.2383980005979538,\n    \"R\": 0.3139890134334564\n   },\n   \"bPrecipitation\": true,\n   \"bWind\": false,\n   \"id\": \"SoftRainSunset\"\n  },\n  {\n   \"CloudColor\": {\n    \"A\": 1.0,\n    \"B\": 0.16145800054073334,\n    \"G\": 0.14209100604057312,\n    \"R\": 0.1269800066947937\n   },\n   \"CloudOpacity\": 1.0,\n   \"Day\": 1,\n   \"FogCutoffDistance\": 0.0,\n   \"FogDensity\": 0.0,\n   \"FogHeightFalloff\": 0.20000000298023224,\n   \"FogInscatteringColor\": {\n    \"A\": 1.0,\n    \"B\": 1.0,\n    \"G\": 0.6380000114440918,\n    \"R\": 0.4449999928474426\n   },\n   \"FogMaxOpacity\": 1.0,\n   \"FogStartDistance\": 0.0,\n   \"HorizonColor\": {\n    \"A\": 1.0,\n    \"B\": 0.010417000390589237,\n    \"G\": 0.010417000390589237,\n    \"R\": 0.0\n   },\n   \"HorizonFalloff\": 10.0,\n   \"Hours\": 12,\n   \"IsDaylightSavingTime\": true,\n   \"Latitude\": 30.237119674682617,\n   \"Longitude\": -97.66307067871094,\n   \"Minutes\": 0,\n   \"Month\": 6,\n   \"NorthOffset\": 0.0,\n   \"OverallSkyColor\": {\n    \"A\": 1.0,\n    \"B\": 0.15625,\n    \"G\": 0.15625,\n    \"R\": 0.15625\n   },\n   \"OverideTimeBasedSunAngle\": true,\n   \"PrecipitationAccumulation\": 0.0,\n   \"PrecipitationAmount\": 0.0,\n   \"PrecipitationType\": \"Rain\",\n   \"SecondFogDensity\": 0.0,\n   \"SecondFogHeightFalloff\": 0.20000000298023224,\n   \"SecondFogHeightOffset\": 0.0,\n   \"Seconds\": 0,\n   \"SkyLightColor\": {\n    \"A\": 255.0,\n    \"B\": 225.0,\n    \"G\": 240.0,\n    \"R\": 247.0\n   },\n   \"SkyLightIntensity\": 0.0,\n   \"StarBrightness\": 0.699999988079071,\n   \"SunAzimuthAngle\": 45.0,\n   \"SunBrightness\": 0.0,\n   \"SunDirectionalLightColor\": {\n    \"A\": 1.0,\n    \"B\": 1.0,\n    \"G\": 1.0,\n    \"R\": 1.0\n   },\n   \"SunDirectionalLightIntensity\": 0.0,\n   \"SunPolarAngle\": 45.0,\n   \"TimeZone\": -5.0,\n   \"WindAngle\": 0.0,\n   \"WindIntensity\": 10.0,\n   \"Year\": 2018,\n   \"ZenithColor\": {\n    \"A\": 1.0,\n    \"B\": 0.004776999820023775,\n    \"G\": 0.004776999820023775,\n    \"R\": 0.0\n   },\n   \"bPrecipitation\": false,\n   \"bWind\": true,\n   \"id\": \"Nighttime\"\n  }\n ],\n \"set_description\": \"Default\"\n}"
  # "Weather Profiles"
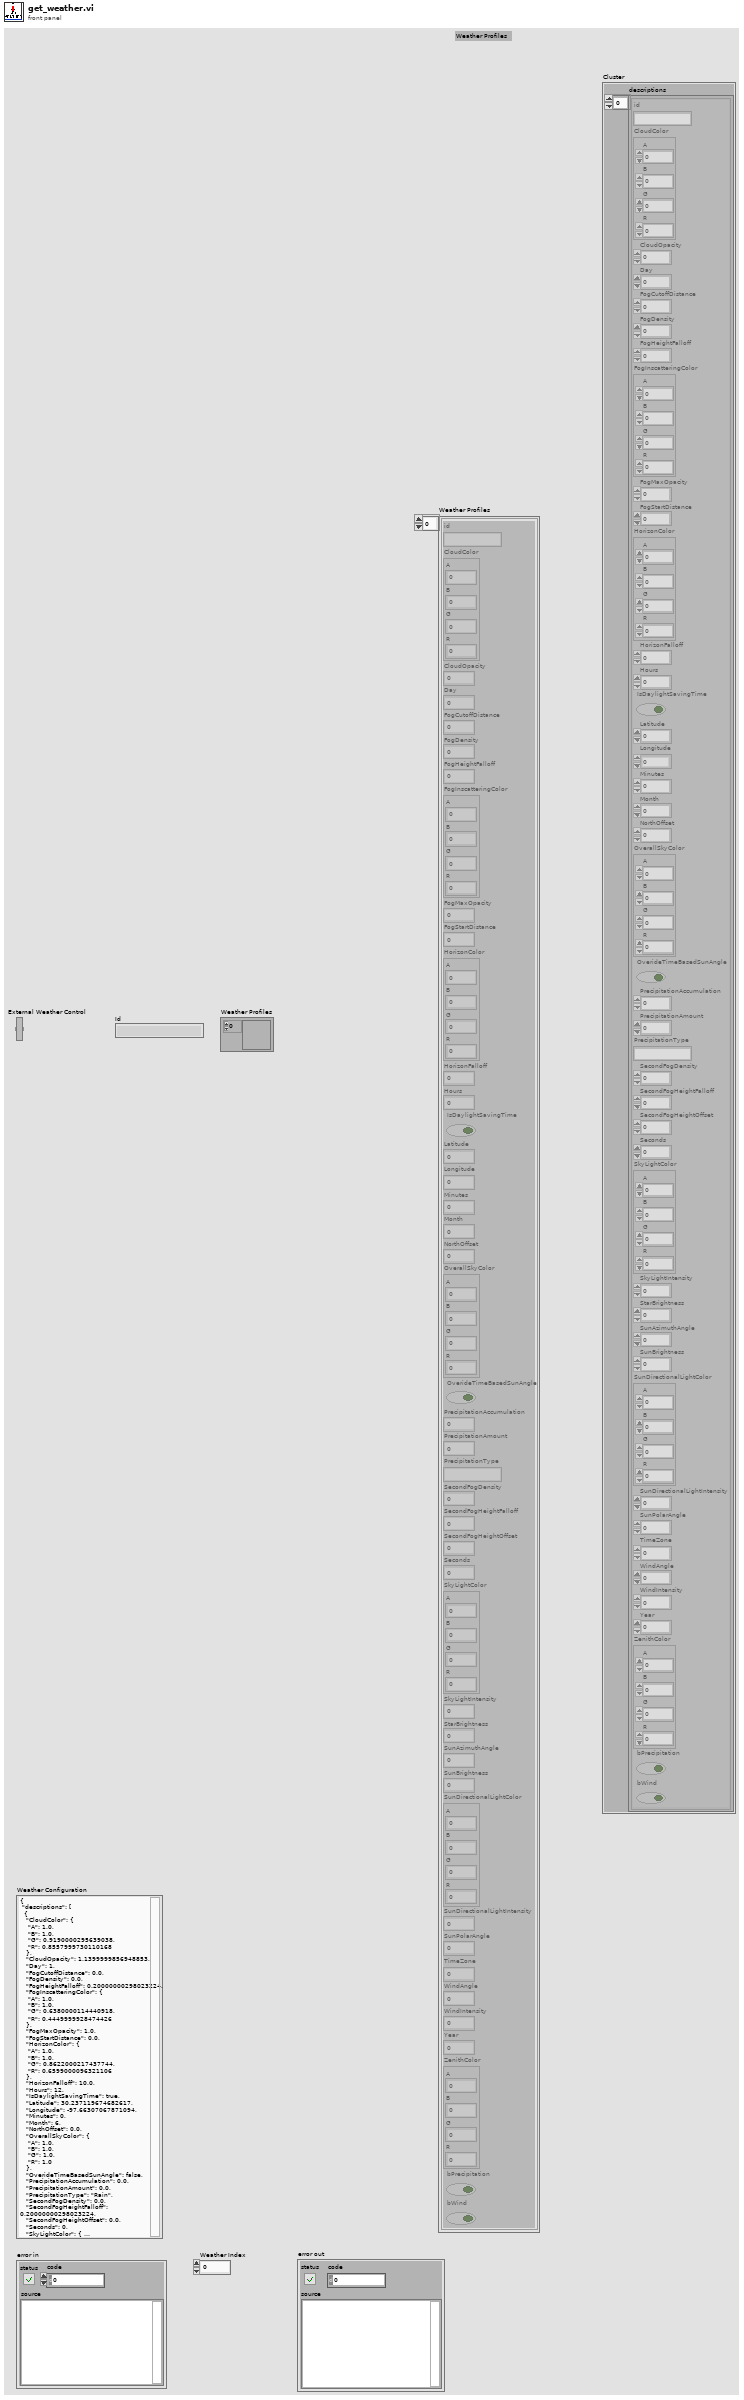
[diagram p1: front panel]
types:
  T1 = cluster{"descriptions":cluster{"id":string, "CloudColor":cluster{"A":sgl, "B":sgl, "G":sgl, "R":sgl}, "CloudOpacity":sgl, "Day":sgl, "FogCutoffDistance":sgl, "FogDensity":sgl, "FogHeightFalloff":sgl, "FogInscatteringColor":cluster{"A":sgl, "B":sgl, "G":sgl, "R":sgl}, "FogMaxOpacity":sgl, "FogStartDistance":sgl, "HorizonColor":cluster{"A":sgl, "B":sgl, "G":sgl, "R":sgl}, "HorizonFalloff":sgl, "Hours":sgl, "IsDaylightSavingTime":bool, "Latitude":sgl, "Longitude":sgl, "Minutes":sgl, "Month":sgl, "NorthOffset":sgl, "OverallSkyColor":cluster{"A":sgl, "B":sgl, "G":sgl, "R":sgl}, "OverideTimeBasedSunAngle":bool, "PrecipitationAccumulation":sgl, "PrecipitationAmount":sgl, "PrecipitationType":string, "SecondFogDensity":sgl, "SecondFogHeightFalloff":sgl, "SecondFogHeightOffset":sgl, "Seconds":sgl, "SkyLightColor":cluster{"A":sgl, "B":sgl, "G":sgl, "R":sgl}, "SkyLightIntensity":sgl, "StarBrightness":sgl, "SunAzimuthAngle":sgl, "SunBrightness":sgl, "SunDirectionalLightColor":cluster{"A":sgl, "B":sgl, "G":sgl, "R":sgl}, "SunDirectionalLightIntensity":sgl, "SunPolarAngle":sgl, "TimeZone":sgl, "WindAngle":sgl, "WindIntensity":sgl, "Year":sgl, "ZenithColor":cluster{"A":sgl, "B":sgl, "G":sgl, "R":sgl}, "bPrecipitation":bool, "bWind":bool}[]}
  T2 = typedef "simx_connection.ctl" = cluster{"Config":T3, "Connections":T6, "Map":cluster{"lanes":cluster{"x":dbl[], "y":dbl[], "z":dbl[]}, "StartPosition":cluster{"start_points":T7, "StartRotation":dbl[], "StartLocation":dbl[]}, "Draw Map Size":T8, "DrawArea":cluster{"min_Y":dbl, "min_X":dbl, "Scale X":dbl, "Scale Y":dbl}, "Map":picture, "Map Geojson":string}}
  T3 = typedef "config.ctl" = cluster{"Trajectory":T4, "Weather":T5}
  T4 = typedef "trajectory.ctl" = cluster{"Number of frames":i32, "Frame number":i32, "Trajectory":string}
  T5 = typedef "weather.ctl" = cluster{"id":string}
  T6 = typedef "connections.ctl" = cluster{"Simulator Connection":refnum<k5>, "server_ip":string, "Port":i32, "Sensor connections":refnum<k5>[]}
  T7 = typedef "start_points.ctl" = cluster{"locations":dbl[][], "rotations":dbl[][], "type":string[]}
  T8 = typedef "LVBoundsTypeDef.ctl" = cluster{"Width":u32, "Height":u32}
  T9 = cluster{"id":string, "CloudColor":cluster{"A":sgl, "B":sgl, "G":sgl, "R":sgl}, "CloudOpacity":sgl, "Day":sgl, "FogCutoffDistance":sgl, "FogDensity":sgl, "FogHeightFalloff":sgl, "FogInscatteringColor":cluster{"A":sgl, "B":sgl, "G":sgl, "R":sgl}, "FogMaxOpacity":sgl, "FogStartDistance":sgl, "HorizonColor":cluster{"A":sgl, "B":sgl, "G":sgl, "R":sgl}, "HorizonFalloff":sgl, "Hours":sgl, "IsDaylightSavingTime":bool, "Latitude":sgl, "Longitude":sgl, "Minutes":sgl, "Month":sgl, "NorthOffset":sgl, "OverallSkyColor":cluster{"A":sgl, "B":sgl, "G":sgl, "R":sgl}, "OverideTimeBasedSunAngle":bool, "PrecipitationAccumulation":sgl, "PrecipitationAmount":sgl, "PrecipitationType":string, "SecondFogDensity":sgl, "SecondFogHeightFalloff":sgl, "SecondFogHeightOffset":sgl, "Seconds":sgl, "SkyLightColor":cluster{"A":sgl, "B":sgl, "G":sgl, "R":sgl}, "SkyLightIntensity":sgl, "StarBrightness":sgl, "SunAzimuthAngle":sgl, "SunBrightness":sgl, "SunDirectionalLightColor":cluster{"A":sgl, "B":sgl, "G":sgl, "R":sgl}, "SunDirectionalLightIntensity":sgl, "SunPolarAngle":sgl, "TimeZone":sgl, "WindAngle":sgl, "WindIntensity":sgl, "Year":sgl, "ZenithColor":cluster{"A":sgl, "B":sgl, "G":sgl, "R":sgl}, "bPrecipitation":bool, "bWind":bool}[]
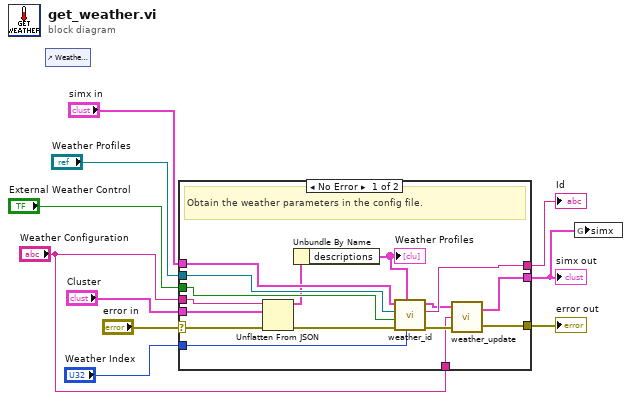
[diagram p0: block diagram]
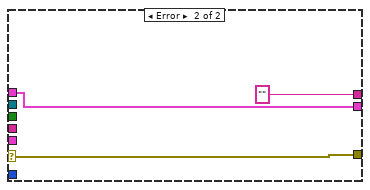
[diagram p2: hidden frame]
diagram:
  n1 = control-ref of="Weather Profiles"() -> ()  [unwired: 1 out]
  n2 = case shown="No Error" "error in" {
    selector: "error in" -> [w20 w29]
    tunnel: [w16 w29] -> w10
    tunnel: "Cluster" -> [w12 _]
    tunnel: "simx in" -> [w21 w28]
    tunnel: "External Weather Control" -> [w26 _]
    tunnel: "Weather Index" -> [w25 _]
    tunnel: [w14 w28] -> w2
    tunnel: [w23 "" ("id")] -> w4
    tunnel: "Weather Profiles" -> [w22 _]
    tunnel: "Weather Configuration" -> [w19 _]
    tunnel: "Weather Configuration" -> [w13 _]
    frame No Error {
      # "Obtain the weather parameters in the config file."
      n3 = Unflatten From JSON(JSON string=w19, type and defaults=w12, error in (no error)=w20) -> (value=w18:T1, error out=w24:errorcluster)  [unwired: 4 in]
      n4 = Unbundle By Name(w18) -> ("descriptions"=w11:T9)
      "Weather Profiles" <- w11
      n5 = call "weather_id.vi"("Weather Index"=w25, 7:"Weather Profiles"=w11, "error in"=w24, "External Weather Control"=w26, 10:"Weather Profiles"=w22, "simx in"=w21) -> ("error out"=w17:errorcluster, "id"=w23:string, "simx out"=w15:T2)  [unwired: 3 in]
      n6 = call "weather_update.vi"("error in"=w17, "Weather Configuration"=w13, "simx in"=w15) -> ("error out"=w16:errorcluster, "simx out"=w14:T2)
    }
    frame Error {
    }
  }
  "error out" <- w10
  "simx out" <- w2
  "Id" <- w4
  n7 = global write "simx_common.vi" "simx"(w2) -> ()
